vi "TrainDriver1.vi"(8 "Horn":bool, 9 "wait":dbl=0.5, 10 "Brake Control":dbl(knob) scale=0.0..1.0, 11 "Throttle Control":dbl(knob)=0.2 scale=-1.0..1.0) -> ()   [LabVIEW 2014]
uses:
  Libraries/Contact Data/Contact.ctl
  Libraries/Contact Data/Position.ctl
  Libraries/Contact Data/Controls.ctl
  Libraries/Contact Data/DestinationCluster.ctl
  Libraries/Contact Data/DesinationControls.ctl
  Libraries/Contact Data/Command.ctl
  Libraries/Contact Data/Contact Data.lvlib
panel:
  in  "milliseconds to wait":u32=250
  in  "stop":bool=TRUE
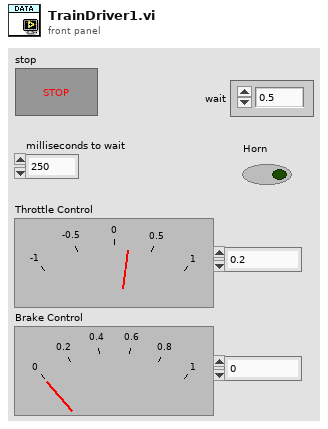
[diagram p1: front panel]
types:
  T1 = typedef "Contact Data.lvlib/Command.ctl" = enum16{"Set All Contacts", "Load", "Save", "Get All Data", "Get Single Data (ID)", "Get Single Data", "Set Position", "Set Destinations", "Set Controls", "Remove Single Data", "Remove UUID Contact", "Set Single ALL", "Is Data Modified", "Import Data"}
  T2 = typedef "Contact Data.lvlib/Contact.ctl" = cluster{"ID":u32, "UUID":string, "Name":string, "Iteration":i32, "Posit Array":T3[], "Controls":T4, "DestArray":T5[], "SetSpeed":dbl, "Speed":dbl}
  T3 = typedef "Contact Data.lvlib/Position.ctl" = cluster{"X":dbl, "Y":dbl, "Z":dbl}
  T4 = typedef "Contact Data.lvlib/Controls.ctl" = cluster{"throttle":dbl, "brake":dbl, "horn":dbl, "wait":dbl}
  T5 = typedef "Contact Data.lvlib/DestinationCluster.ctl" = cluster{"Desination":string, "DestControls":T6, "Timer":u32, "Set Timer":u32, "Time Stamp":timestamp, "Repeat?":bool, "Optional Data":string, "Distance":dbl}
  T6 = typedef "Contact Data.lvlib/DesinationControls.ctl" = enum16{"Tracker", "Manual", "Stop", "Station DateTime", "Station Timer", "Maintain"}
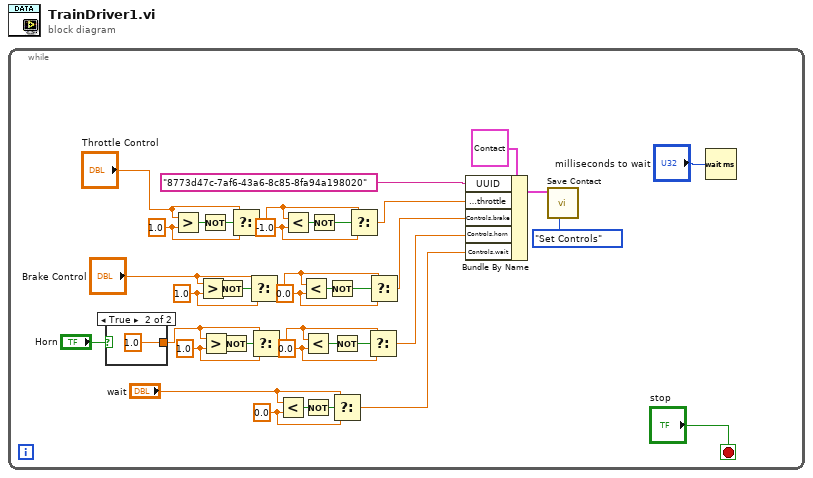
[diagram p0: block diagram]
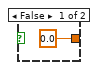
[diagram p2: hidden frame]
diagram:
  n1 = while {
    stop <- "stop" stop-if-true
    w20 = 0.0 ("y")
    w23 = 0.0 ("y")
    w24 = 1.0 ("y")
    w28 = 0.0 ("y")
    w27 = 1.0 ("y")
    w32 = -1.0 ("y")
    w33 = 1.0 ("y")
    n2 = case shown="True" "Horn" {
      tunnel: [0.0 ("y") 1.0 ("y")] -> w2
      frame False {
      }
      frame True {
      }
    }
    n3 = Greater?(x="Throttle Control", y=w33) -> (0:w34:bool)
    n4 = Greater?(x="Brake Control", y=w27) -> (0:w26:bool)
    n5 = Not(x=w34) -> (.not. x?=w6:bool)
    n6 = Greater?(x=w2, y=w24) -> (0:w25:bool)
    n7 = Not(x=w26) -> (.not. x?=w8:bool)
    n8 = Not(x=w25) -> (.not. x?=w11:bool)
    n9 = Select(t="Throttle Control", s=w6, f=w33) -> (s? t:f=w14:dbl)
    n10 = Select(t="Brake Control", s=w8, f=w27) -> (s? t:f=w15:dbl)
    n11 = Select(t=w2, s=w11, f=w24) -> (s? t:f=w13:dbl)
    n12 = Less?(x="wait", y=w20) -> (x < y?=w21:bool)
    n13 = Less?(x=w14, y=w32) -> (x < y?=w31:bool)
    n14 = Less?(x=w15, y=w28) -> (x < y?=w29:bool)
    n15 = Less?(x=w13, y=w23) -> (x < y?=w22:bool)
    n16 = Not(x=w21) -> (.not. x?=w12:bool)
    n17 = Not(x=w31) -> (.not. x?=w7:bool)
    n18 = Not(x=w29) -> (.not. x?=w9:bool)
    n19 = Not(x=w22) -> (.not. x?=w10:bool)
    n20 = Select(t="wait", s=w12, f=w20) -> (s? t:f=w19:dbl)
    n21 = Select(t=w14, s=w7, f=w32) -> (s? t:f=w30:dbl)
    n22 = Select(t=w13, s=w10, f=w23) -> (s? t:f=w17:dbl)
    n23 = Select(t=w15, s=w9, f=w28) -> (s? t:f=w16:dbl)
    n24 = Bundle By Name(cluster=T2 {"ID"=0, "UUID"="", "Name"="", "Iteration"=0, "Posit Array"=[], "Controls"={"throttle"=0.0, "brake"=0.0, "horn"=0.0, "wait"=0.5}, "DestArray"=[], "SetSpeed"=0.0, "Speed"=0.0} ("Contact"), "UUID"="8773d47c-7af6-43a6-8c85-8fa94a198020", "Controls.throttle"=w30, "Controls.brake"=w16, "Controls.horn"=w17, "Controls.wait"=w19) -> (w38:T2)
    n25 = call "Save Contact.vi"("Command"=Command."Set Controls", "Contact"=w38) -> ()  [unwired: 8 in, 2 out]
    n26 = Wait (ms)(milliseconds to wait="milliseconds to wait") -> ()  [unwired: 1 out]
  }
